vi "Ramp Create Ramp Array Based on # of Elements.vi"(0 "Initial Value (0.0)":dbl format="%.2f", 7 "Final Value (0.0)":dbl format="%.2f", 11 "# of Elements (0)":i32) -> (4 "Output Array":dbl[](array[numeric]) format="%.2f", 15 "Step Size":dbl format="%.6f")   [LabVIEW 2018]
doc: "Creates a ramp array from an initial value to a final value with the specified # of elements. \n\nIf # of elements < 1: output array is empty.\nIf # of elements = 1: output array is single element array of initial value.\nIf # of elements > 1: otuput array has the specified number of elements, with values evenly spaced between (and including) the initial and final values.\n\nThis VI is similar to the built-in LabVIEW function \"Ramp Pattern.vi\", except that support for a single-element array has been added."
uses:
  <vilib>/Analysis/1siggen.llb/Ramp Pattern by Samples.vi
  <vilib>/Analysis/NI_AALBase.lvlib
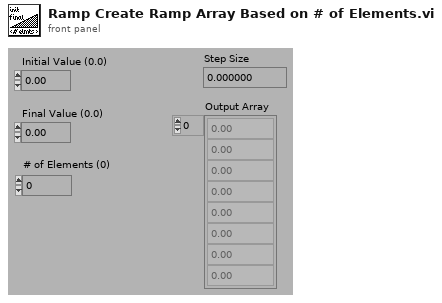
[diagram p1: front panel]
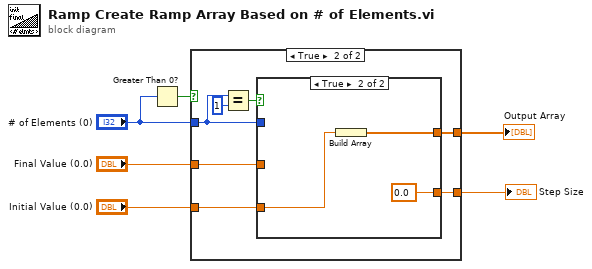
[diagram p0: block diagram]
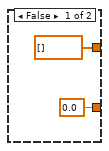
[diagram p2: hidden frame]
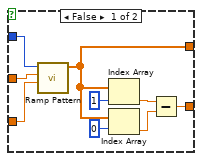
[diagram p3: hidden frame]
diagram:
  n1 = Greater Than 0?(x="# of Elements (0)") -> (x > 0?=w2:bool)
  n2 = case shown="True" w2 {
    tunnel: [dbl[] [] ("Ramp Pattern") w15] -> w4
    tunnel: "# of Elements (0)" -> [_ w12]
    tunnel: "Initial Value (0.0)" -> [_ w14]
    tunnel: "Final Value (0.0)" -> [_ w13]
    tunnel: [0.0 w9] -> w1
    frame False {
    }
    frame True {
      n3 = Equal?(x=w12, y=1) -> (x = y?=w10:bool)
      n4 = case shown="True" w10 {
        tunnel: w13 -> [w24 _]
        tunnel: w14 -> [w23 w27]
        tunnel: w12 -> [w22 _]
        tunnel: [w21 w26] -> w15
        tunnel: [w16 0.0] -> w9
        frame False {
          n5 = call-poly <vilib>:"Ramp Pattern.vi"("start"=w23, "end"=w24, "samples"=w22) -> ("Ramp Pattern"=w21:dbl[])  [unwired: 7 in, 1 out]
          n6 = Index Array(array=w21, index=1) -> (element=w18:dbl)
          n7 = Index Array(array=w21, index=0) -> (element=w17:dbl)
          n8 = Subtract(x=w18, y=w17) -> (x-y=w16:dbl)
        }
        frame True {
          n9 = Build Array(w27) -> (w26:dbl[])
        }
      }
    }
  }
  "Output Array" <- w4
  "Step Size" <- w1
